vi "get_shape.vi"(8 "error in (no error)":errorcluster caption="entrée d'erreur (pas d'erreur)", 11 "SpectralCoclustering.lvclass":refnum<class "SpectralCoclustering.lvclass">) -> (0 "error out":errorcluster caption="sortie d'erreur", 2 "out":cluster{"n_rows":dbl, "n_cols":dbl}, 3 "SpectralCoclustering.lvclass 2":refnum<class "SpectralCoclustering.lvclass">)   [LabVIEW 2020, in "SpectralCoclustering.lvclass"]
doc: "Shape of the i’th bicluster."
uses:
  SpectralCoclustering.lvclass
  C:/Users/cipop/TDF Dropbox/2_Technologies de France/1 - Services et Etudes/PLAIY/2 - DEV/PLAIYLAB/code/Python/Python.lvclass
  C:/Users/cipop/TDF Dropbox/2_Technologies de France/1 - Services et Etudes/PLAIY/2 - DEV/PLAIYLAB/code/Model/Model.lvclass
  SpectralCoclustering.lvclass/SpectralCoclustering.ctl
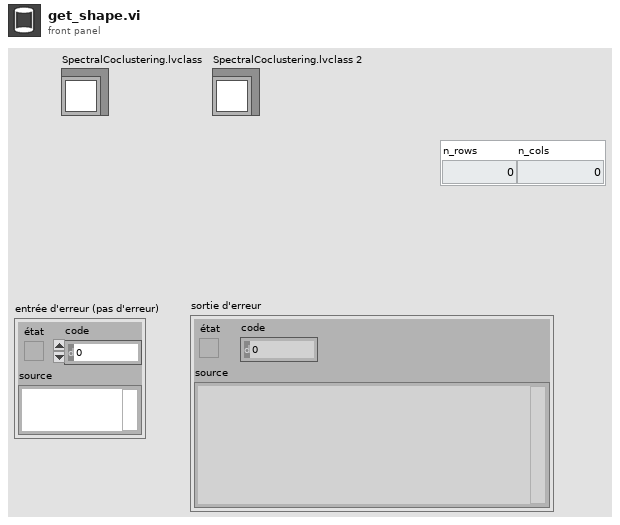
[diagram p1: front panel]
types:
  T1 = typedef "data.ctl" = cluster{"name":string, "X":dbl[][]}
  T2 = typedef "spectral_coclustering_data.ctl" = cluster{"i":dbl, "data":dbl[][]}
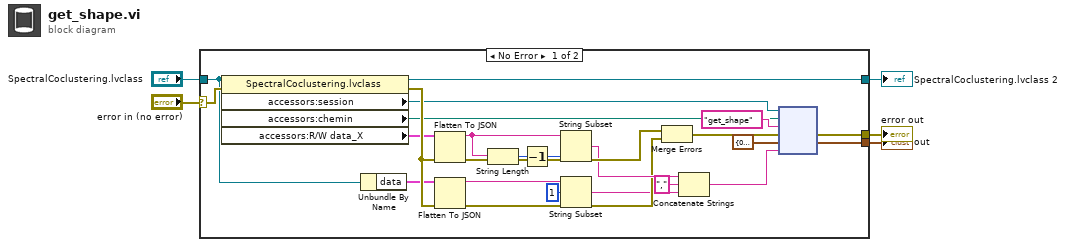
[diagram p0: block diagram]
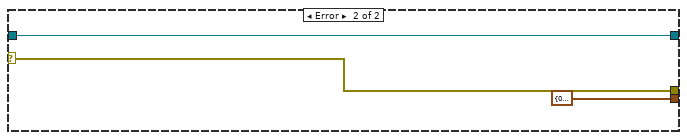
[diagram p2: hidden frame]
diagram:
  n1 = case shown="No Error" "error in (no error)" {
    selector: "error in (no error)" -> [w27 w32]
    tunnel: [w28 w32] -> w2
    tunnel: [w8 w31] -> w3
    tunnel: "SpectralCoclustering.lvclass" -> [w7 w31]
    tunnel: [w13 cluster{"row_ind":dbl, "col_ind":dbl} {"row_ind"=0.0, "col_ind"=0.0} ("out")] -> w1
    frame No Error {
      n2 = property class="SpectralCoclustering.lvclass"(reference=w7, error in=w27) -> (reference out=w8:refnum<class "SpectralCoclustering.lvclass">, error out=w18:errorcluster, "accessors:session"=w10:refnum<k35>, "accessors:chemin"=w9:path, "accessors:R/W data_X"=w12:T1)
      n3 = Unbundle By Name(w7) -> ("data"=w6:T2)
      n4 = Flatten To JSON(anything=w12, error in (no error)=w18) -> (JSON string=w24:string, 11:w21:errorcluster)  [unwired: 1 in]
      n5 = Flatten To JSON(anything=w6, error in (no error)=w18) -> (JSON string=w22:string, 11:w17:errorcluster)  [unwired: 1 in]
      n6 = String Length(string=w24) -> (length=w26:i32)
      n7 = Decrement(x=w26) -> (x-1=w25:i32)
      n8 = String Subset(string=w24, length (rest)=w25) -> (substring=w20:string)  [unwired: 1 in]
      n9 = String Subset(string=w22, offset (0)=1) -> (substring=w15:string)  [unwired: 1 in]
      n10 = Merge Errors(w21, w17) -> (w11:errorcluster)
      n11 = Concatenate Strings(w20, "," ("string"), w15) -> (w19:string)
      n12 = node(w10, w9, "get_shape" ("nom de la fonction"), w11, cluster{"row_ind":dbl, "col_ind":dbl} {"row_ind"=0.0, "col_ind"=0.0} ("out"), w19) -> (w28:errorcluster, w13:cluster{"row_ind":dbl, "col_ind":dbl})  [unwired: 1 in, 3 out]
    }
    frame Error {
    }
  }
  "error out" <- w2
  "SpectralCoclustering.lvclass 2" <- w3
  "out" <- w1
